vi "Change Endianness (U32).vi"(11 "number in":u32) -> (3 "byte-reversed number out":u32)   [LabVIEW 2016, in "GE 5565PIORC Old.lvclass"]
uses:
  GE 5565PIORC Old.lvclass
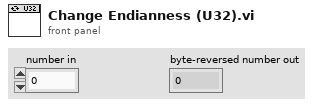
[diagram p1: front panel]
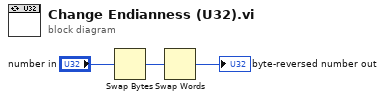
[diagram p0: block diagram]
diagram:
  n1 = Swap Bytes(anything="number in") -> (byte swapped=w2:u32)
  n2 = Swap Words(1:w2) -> (0:→"byte-reversed number out":u32)
